vi "Read TDMS Channel-Group Names.vi"(8 "error in":errorcluster, 11 "File Path Control":path) -> (0 "error out":errorcluster, 2 "File-group-channel":T1[](array[typedef]))   [LabVIEW 2021]
uses:
  File_Group_Chan_Abbr.ctl
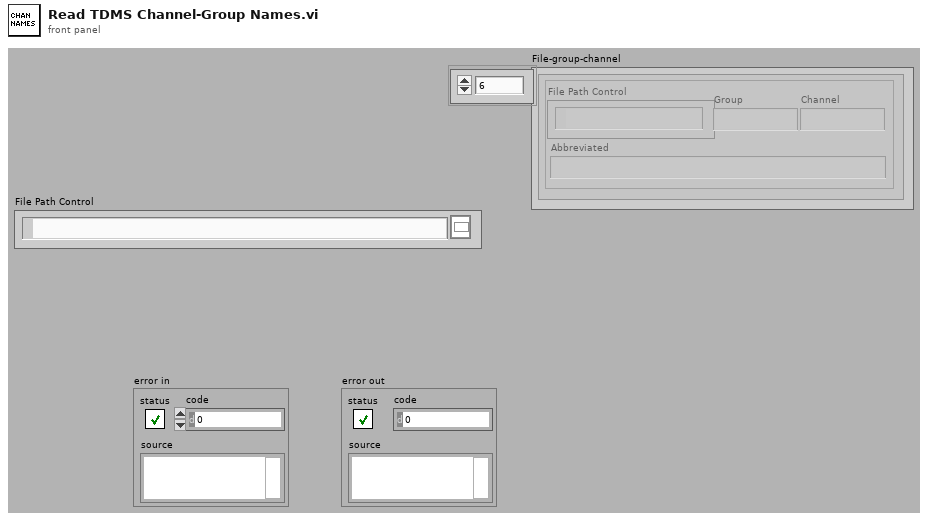
[diagram p1: front panel]
types:
  T1 = typedef "File_Group_Chan_Abbr.ctl" = cluster{"File Path Control":path, "Group":string, "Channel":string, "Abbreviated":string}
  T2 = enum16{"open", "open or create", "create or replace", "create", "open (read-only)"}
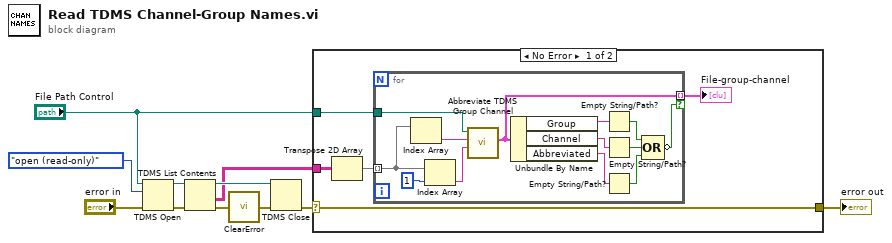
[diagram p0: block diagram]
diagram:
  n1 = TDMS Open(8:"error in", 10:T2."open (read-only)" ("operation (0:open)"), 11:"File Path Control") -> (0:w9:errorcluster, 3:w8:refnum<k34>)  [unwired: 4 in]
  n2 = TDMS List Contents(4:w9, 7:w8) -> (0:w1:errorcluster, 1:w5:string[][], 3:w7:refnum<k34>)  [unwired: 2 out]
  n3 = call <vilib>:"ClearError.vi"("error in (no error)"=w1) -> ("error out"=w6:errorcluster)
  n4 = TDMS Close(8:w6, 11:w7) -> (0:w3:errorcluster)  [unwired: 1 out]
  n5 = case shown="No Error" w3 {
    selector: w3 -> [w12 w30]
    tunnel: w5 -> [w16 _]
    tunnel: "File Path Control" -> [w13 _]
    tunnel: [w12 w30] -> w2
    frame No Error {
      n6 = Transpose 2D Array(2D array=w16) -> (transposed array=w14:string[][])
      n7 = for {
        tunnel: w14 -> [w29] mode=indexing
        tunnel: w13 -> [w25]
        tunnel: [w19] -> w15 mode=indexing if=w26
        n8 = Index Array(array=w29) -> (element=w21:string)  [unwired: 1 in]
        n9 = Index Array(array=w29, index=1) -> (element=w20:string)
        n10 = call "Abbreviate TDMS Group Channel.vi"("Channel"=w20, "Group"=w21, "File Path Control"=w25) -> ("Cluster"=w19:T1)  [unwired: 7 in, 1 out]
        n11 = Unbundle By Name(w19) -> ("Group"=w24:string, "Channel"=w23:string, "Abbreviated"=w22:string)
        n12 = Empty String/Path?(string/path=w24) -> (empty?=w17:bool)
        n13 = Empty String/Path?(string/path=w23) -> (empty?=w27:bool)
        n14 = Empty String/Path?(string/path=w22) -> (empty?=w18:bool)
        n15 = Compound Arithmetic op=OR(w17, w27, w18) -> (invert w26:bool)
      }
      "File-group-channel" <- w15
    }
    frame Error {
    }
  }
  "error out" <- w2
